vi "Part 1.vi"() -> ()   [LabVIEW 2016]
panel:
  in  "Boolean 2":bool
  in  "stop":bool
  out "Boolean":bool
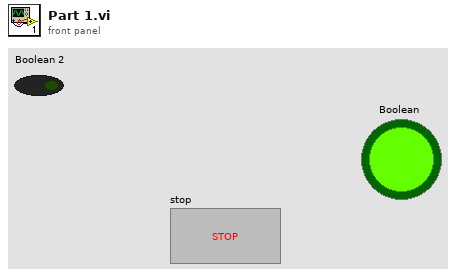
[diagram p1: front panel]
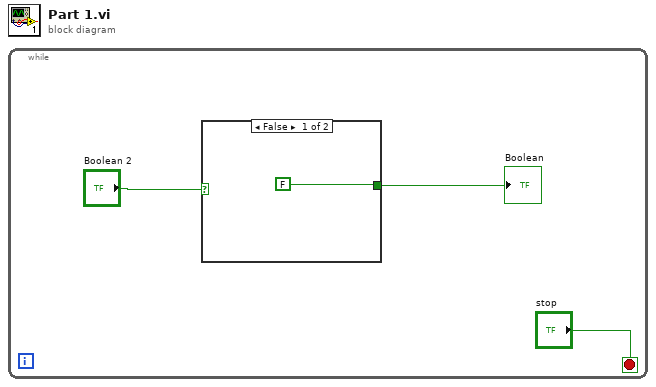
[diagram p0: block diagram]
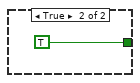
[diagram p2: hidden frame]
diagram:
  n1 = while {
    stop <- "stop" stop-if-true
    n2 = case shown="False" "Boolean 2" {
      tunnel: [FALSE TRUE] -> w3
      frame False {
      }
      frame True {
      }
    }
    "Boolean" <- w3
  }
